vi "DynamicLoadLRvi.vi"(0 "LibName\\viName":string="CRC与诊断.lvlibp\\CRC与诊断\\CRC类\\CRC计算.vi", 1 "校验算法名称":string="Anti_Add", 2 "校验数据":u8[](array[numeric])=[215, 130, 0, 0, 0, 0, 11, 0] format="%x", 3 "校验长度":u8=7) -> (14 "校验值":u64=7)   [LabVIEW 2020]
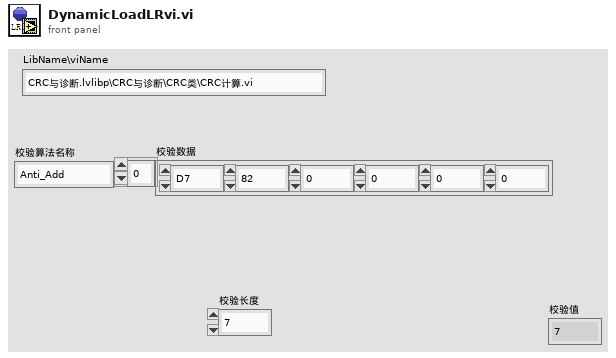
[diagram p1: front panel]
types:
  T1 = enum32{"invalid app kind", "Development System", "Run Time System", "Student Edition", "Embedded LabVIEW", "Evaluation", "Custom"}
  T2 = enum32{"Invalid", "Standard", "Closed", "Hidden", "Minimized", "Maximized"}
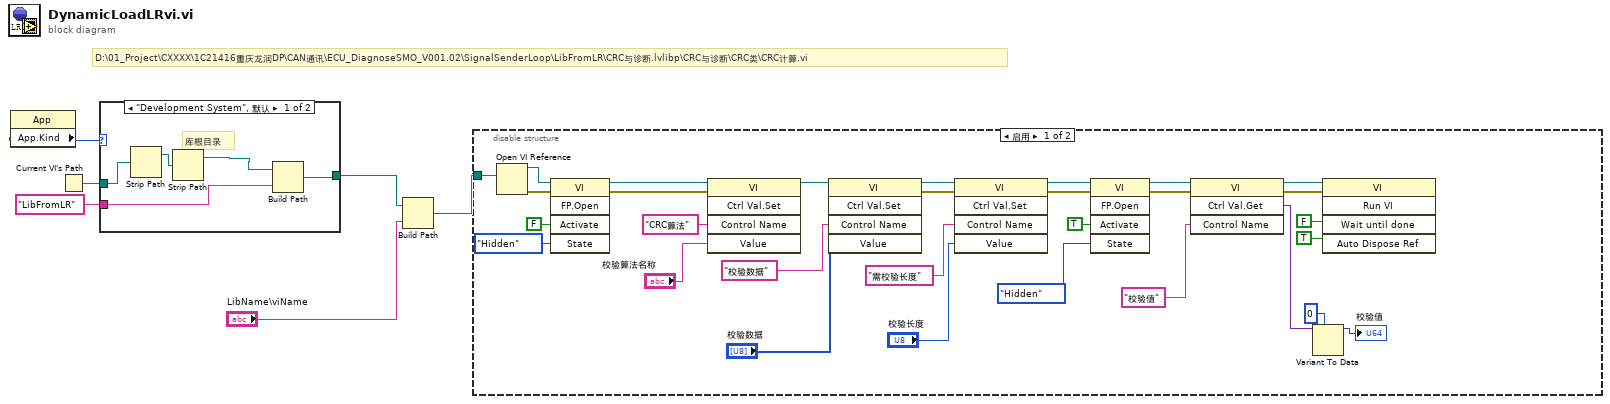
[diagram p0: block diagram]
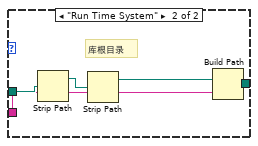
[diagram p3: hidden frame]
diagram:
  # "D:\\01_Project\\CXXXX\\1C21416重庆龙润DP\\CAN通讯\\ECU_DiagnoseSMO_V001.02\\SignalSenderLoop\\LibFromLR\\CRC与诊断.lvlibp\\CRC与诊断\\CRC类\\CRC计算.vi"
  n1 = property class="App"() -> ("App.Kind"=w4:T1)  [unwired: 2 in, 2 out]
  n2 = Current VI's Path() -> (path=w5:path)
  n3 = case shown="\"Development System\", 默认" w4 {
    tunnel: w5 -> [w11 w16]
    tunnel: [w8 w12] -> w3
    tunnel: "LibFromLR" ("ConfigFlieFolderName") -> [w7 w13]
    frame "Development System", Default {
      # "库根目录"
      n4 = Strip Path(path=w11) -> (stripped path=w10:path)  [unwired: 1 out]
      n5 = Strip Path(path=w10) -> (stripped path=w9:path)  [unwired: 1 out]
      n6 = Build Path(base path=w9, name or relative path=w7) -> (appended path=w8:path)
    }
    frame "Run Time System" {
      # "库根目录"
      n7 = Strip Path(path=w16) -> (stripped path=w15:path)  [unwired: 1 out]
      n8 = Strip Path(path=w15) -> (stripped path=w14:path)  [unwired: 1 out]
      n9 = Build Path(base path=w14, name or relative path=w13) -> (appended path=w12:path)
    }
  }
  n10 = Build Path(base path=w3, name or relative path="LibName\\viName") -> (appended path=w1:path)
  n11 = disable-structure shown="启用" {
    disable-tunnel: w1 -> [w34 _]
    frame Enabled {
      n12 = Open VI Reference(vi path=w34) -> (vi reference=w45:refnum<vi>, error out=w46:errorcluster)  [unwired: 5 in]
      n13 = invoke class="VI" method="FP.Open"(reference=w45, error in=w46, "Activate"=FALSE ("激活？"), "State"=T2."Hidden" ("状态")) -> (reference out=w41:refnum<vi>, error out=w44:errorcluster)  [unwired: 1 in, 3 out]
      n14 = invoke class="VI" method="Ctrl Val.Set"(reference=w41, error in=w44, "Control Name"="CRC算法" ("控件名"), "Value"="校验算法名称") -> (reference out=w32:refnum<vi>)  [unwired: 1 in, 4 out]
      n15 = invoke class="VI" method="Ctrl Val.Set"(reference=w32, "Control Name"="校验数据" ("控件名"), "Value"="校验数据") -> (reference out=w31:refnum<vi>, error out=w30:errorcluster)  [unwired: 2 in, 3 out]
      n16 = invoke class="VI" method="Ctrl Val.Set"(reference=w31, error in=w30, "Control Name"="需校验长度" ("控件名"), "Value"="校验长度") -> (reference out=w27:refnum<vi>, error out=w26:errorcluster)  [unwired: 1 in, 3 out]
      n17 = invoke class="VI" method="FP.Open"(reference=w27, error in=w26, "Activate"=TRUE ("激活？"), "State"=T2."Hidden" ("状态")) -> (reference out=w40:refnum<vi>, error out=w39:errorcluster)  [unwired: 1 in, 3 out]
      n18 = invoke class="VI" method="Ctrl Val.Get"(reference=w40, error in=w39, "Control Name"="校验值" ("控件名")) -> (reference out=w38:refnum<vi>, error out=w37:errorcluster, "Get Control Value Variant"=w20:variant)  [unwired: 1 in, 1 out]
      n19 = Variant To Data(type=u64 0 ("校验值"), Variant=w20) -> (data=→"校验值":u64)  [unwired: 1 in, 1 out]
      n20 = invoke class="VI" method="Run VI"(reference=w38, error in=w37, "Wait until done"=FALSE ("Wait Until Done"), "Auto Dispose Ref"=TRUE ("Auto Dispose Reference")) -> ()  [unwired: 1 in, 5 out]
    }
    frame Disabled {
    }
  }
